vi "Launch Analog Input.vi"(8 "error in (no error)":errorcluster, 11 "Top Level in":refnum<class "Top Level.lvclass">) -> (0 "error out":errorcluster, 3 "Top Level out":refnum<class "Top Level.lvclass">)   [LabVIEW 2021, in "Top Level.lvlib" / "Top Level.lvclass"]
uses:
  Top Level.lvclass
  C:/Program Files/National Instruments/LabVIEW 2021/vi.lib/ActorFramework/Actor/Actor.lvclass
  <vilib>/NathanCo/Analog Tasks/Utilities/Analog Configuration Parameters.ctl
  Top Level.lvclass/Top Level.ctl
  <vilib>/NathanCo/Analog Tasks/Analog Input/Analog Input/Analog Input/Analog Input.lvclass
  <vilib>/ActorFramework/Actor/Actor.lvclass
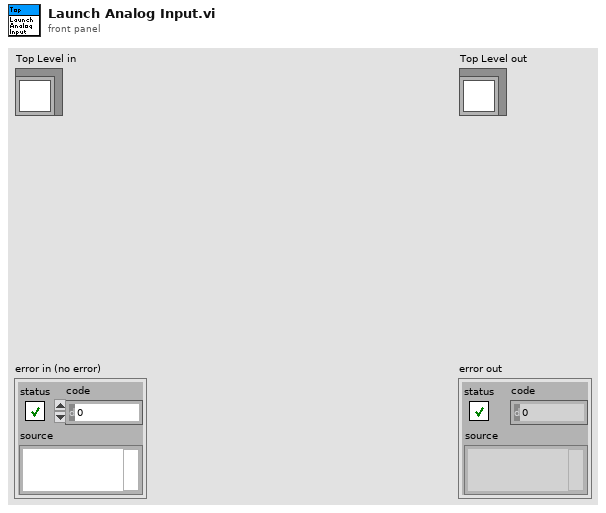
[diagram p1: front panel]
types:
  T1 = typedef "Analog Configuration Parameters.ctl" = cluster{"Terminal Configuration":i32, "Minimum Voltage":dbl, "Maximum Voltage":dbl, "Simulated?":bool, "Device":string, "Device Number":string, "Channel":string, "NI_ChannelName":string}
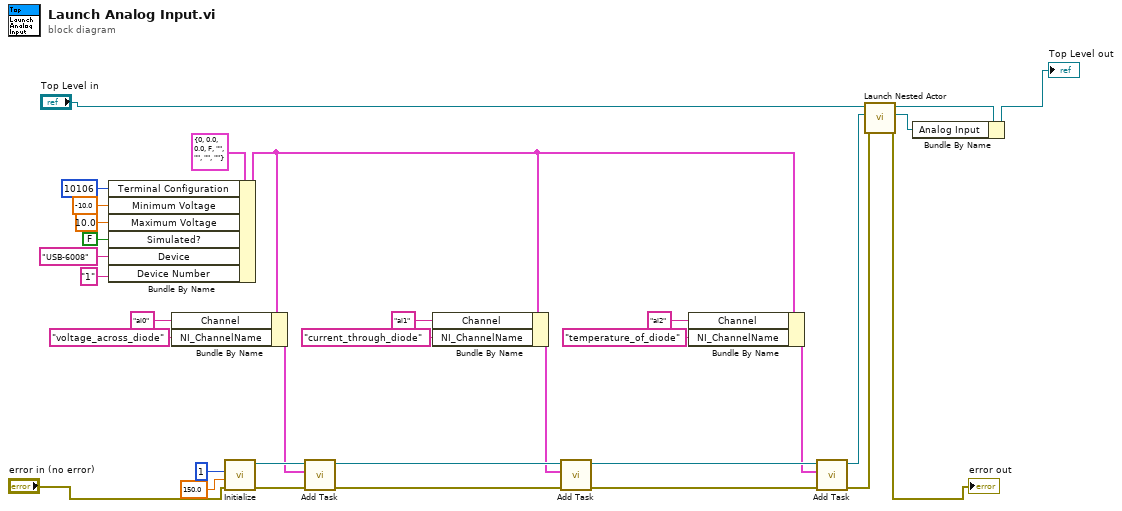
[diagram p0: block diagram]
diagram:
  n1 = Bundle By Name(cluster=T1 {"Terminal Configuration"=0, "Minimum Voltage"=0.0, "Maximum Voltage"=0.0, "Simulated?"=FALSE, "Device"="", "Device Number"="", "Channel"="", "NI_ChannelName"=""} ("Analog Configuration Parameters"), "Terminal Configuration"=10106, "Minimum Voltage"=-10.0, "Maximum Voltage"=10.0, "Simulated?"=FALSE, "Device"="USB-6008", "Device Number"="1") -> (w15:T1)
  n2 = Bundle By Name(cluster=w15, "Channel"="ai0", "NI_ChannelName"="voltage_across_diode") -> (w12:T1)
  n3 = call <vilib>:"Initialize.vi"("error in (no error)"="error in (no error)", "Rate"=150.0, "Number Of Samples Per Channel"=1) -> ("error out"=w26:errorcluster, "Analog Input out"=w31:refnum<class "Analog Input.lvclass">)  [unwired: 7 in]
  n4 = call <vilib>:"Add Task.vi"("error in (no error)"=w26, "Analog Configuration Parameters"=w12, "Analog Input in"=w31) -> ("error out"=w27:errorcluster, "Analog Input out"=w30:refnum<class "Analog Input.lvclass">)  [unwired: 7 in]
  n5 = Bundle By Name(cluster=w15, "Channel"="ai1", "NI_ChannelName"="current_through_diode") -> (w13:T1)
  n6 = call <vilib>:"Add Task.vi"("error in (no error)"=w27, "Analog Configuration Parameters"=w13, "Analog Input in"=w30) -> ("error out"=w28:errorcluster, "Analog Input out"=w29:refnum<class "Analog Input.lvclass">)  [unwired: 7 in]
  n7 = Bundle By Name(cluster=w15, "Channel"="ai2", "NI_ChannelName"="temperature_of_diode") -> (w14:T1)
  n8 = call <vilib>:"Add Task.vi"("error in (no error)"=w28, "Analog Configuration Parameters"=w14, "Analog Input in"=w29) -> ("error out"=w25:errorcluster, "Analog Input out"=w32:refnum<class "Analog Input.lvclass">)  [unwired: 7 in]
  n9 = call <vilib>:"Launch Nested Actor.vi"("error in (no error)"=w25, "Nested Actor"=w32, "Caller Actor in"="Top Level in") -> ("error out"=→"error out":errorcluster, "Nested Actor's Enqueuer"=w5:refnum<class "Message Enqueuer.lvclass">, "Caller Actor out"=w33:refnum<class "Top Level.lvclass">)  [unwired: 6 in]
  n10 = Bundle By Name(cluster=w33, "Analog Input"=w5) -> (→"Top Level out":refnum<class "Top Level.lvclass">)
